vi "AuMT8852B Copy Dirty Table to Loopback Test.vi"(5 "Test (Single-slot sensitivity)":T1(ring), 7 "Script (3)":i32=3, 8 "error in (no error)":errorcluster, 11 "VISA session":refnum<visa-resource-name>) -> (0 "error out":errorcluster, 2 "error code":i32, 3 "VISA session out":refnum<visa-resource-name>)   [LabVIEW 2017]
doc: "Anritsu MT8852B Bluetooth Tester\n\nThis command will configure the set of dirty parameters to be used for the auxiliary loop back command if the dirty transmitter support is enabled. The command selects a dirty parameter table from either the multi slot or single slot sensitivity tests from any script.\n\nINPUTS\nScript - the script to access\nTest - the test from which the values will be copied"
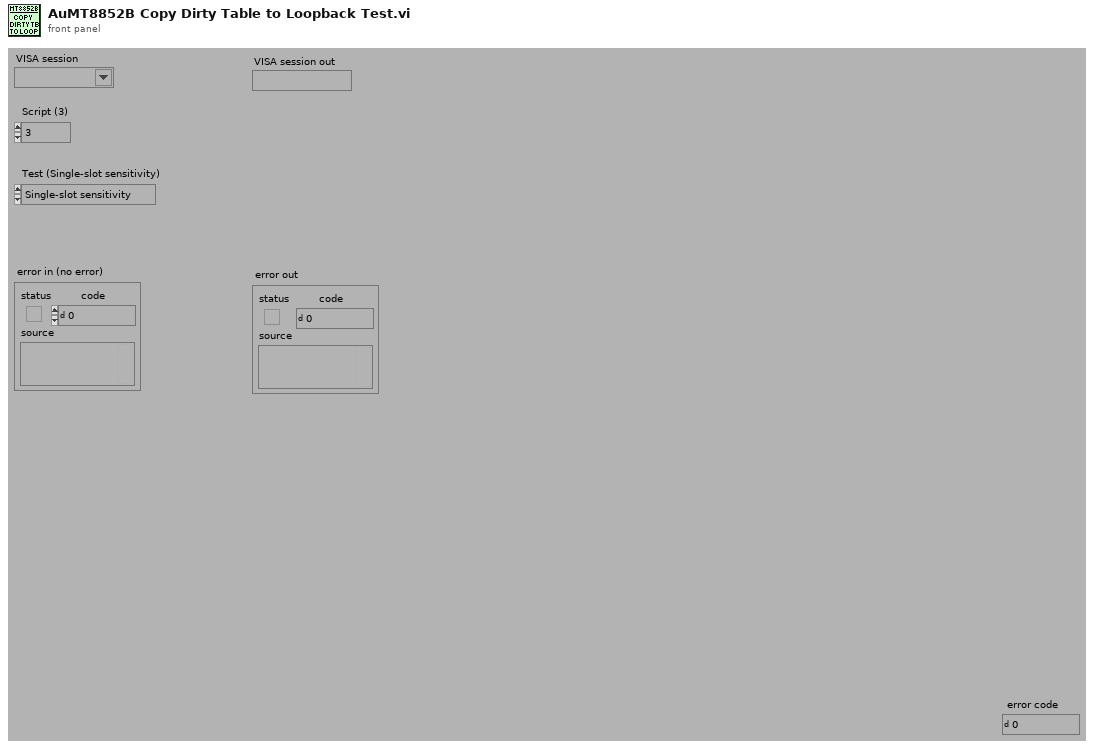
[diagram p1: front panel]
types:
  T1 = enum16{"Single-slot sensitivity", "Multiple-slot sensitivity"}
  T2 = enum16{"Simulate", "Range check", "Cache", "Query instrument status"}
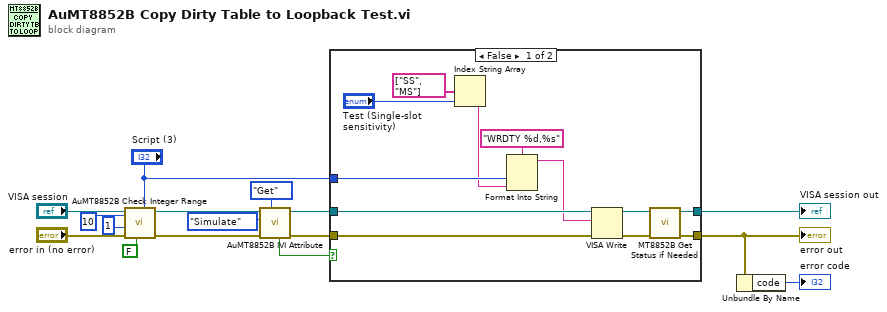
[diagram p0: block diagram]
diagram:
  n1 = call <instrlib>:"AuMT8852B Check Integer Range.vi"("Value (0)"="Script (3)", "Check IVI flag first? (T)"=FALSE, "error in (no error)"="error in (no error)", "Lower limit (-1)"=1, "Upper limit (1)"=10, "VISA session"="VISA session") -> ("error out"=w9:errorcluster, "VISA session out"=w12:refnum<visa-resource-name>)  [unwired: 4 in]
  n2 = call <instrlib>:"AuMT8852B IVI Attribute.vi"("Set/Get (Set)"=enum16{"Set", "Get"}."Get", "error in (no error)"=w9, "Flag (Simulate)"=T2."Simulate", "VISA session"=w12) -> ("error out"=w10:errorcluster, "VISA session out"=w11:refnum<visa-resource-name>, "Value out"=w6:bool)  [unwired: 5 in]
  n3 = case shown="False" w6 {
    tunnel: [w23 w29] -> w3
    tunnel: [w24 w30] -> w16
    tunnel: w11 -> [w28 w30]
    tunnel: w10 -> [w27 w29]
    tunnel: "Script (3)" -> [w22 _]
    frame False {
      n4 = Index String Array(1:"Test (Single-slot sensitivity)", 2:string[] ["SS", "MS"] ("Array Constant")) -> (0:w18:string)  [unwired: 1 in]
      n5 = Format Into String(format string="WRDTY %d,%s" ("Format String"), w22, w18) -> (resulting string=w19:string)  [unwired: 2 in, 1 out]
      n6 = VISA Write(VISA resource name=w28, write buffer=w19, error in (no error)=w27) -> (VISA resource name out=w26:refnum<visa-resource-name>, error out=w25:errorcluster)  [unwired: 1 out]
      n7 = call <instrlib>:"MT8852B Get Status if Needed.vi"("error in (no error)"=w25, "VISA session"=w26) -> ("error out"=w23:errorcluster, "VISA session out"=w24:refnum<visa-resource-name>)  [unwired: 8 in]
    }
    frame True {
    }
  }
  "error out" <- w3
  "VISA session out" <- w16
  n8 = Unbundle By Name(w3) -> ("code"=→"error code":i32)
